vi "AI-Volt.vi"(6 "Slot":T1, 8 "error in":errorcluster, 10 "Mode":string, 11 "CH":string) -> (0 "error out":errorcluster, 3 "data":dbl caption="数据" format="%0.2f")   [LabVIEW 2013]
uses:
  SystemCode/SysControl/Slot.ctl
  <vilib>/DAQmx/read.llb/DAQmx Read (Analog 1D DBL 1Chan NSamp).vi
  SourceCode/GlobalValue.vi
  <vilib>/DAQmx/create/channels.llb/DAQmx Create Channel (AI-Voltage-Basic).vi
  <vilib>/measure/madcrms.llb/Basic Averaged DC-RMS for 1 Chan.vi
  <vilib>/DAQmx/miscellaneous.llb/DAQmx Fill In Error Info.vi
  <vilib>/measure/NI_MAPro.lvlib
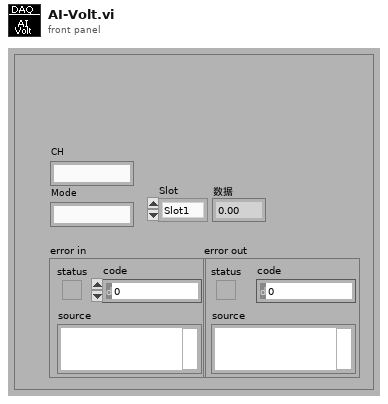
[diagram p1: front panel]
types:
  T1 = typedef "Slot.ctl" = enum16{"Slot1", "Slot2", "Slot3", "Slot4"}
  T2 = typedef "DAQConfig.ctl" = cluster{"DIO":string[][], "AO":string[][], "AI":string[][]}
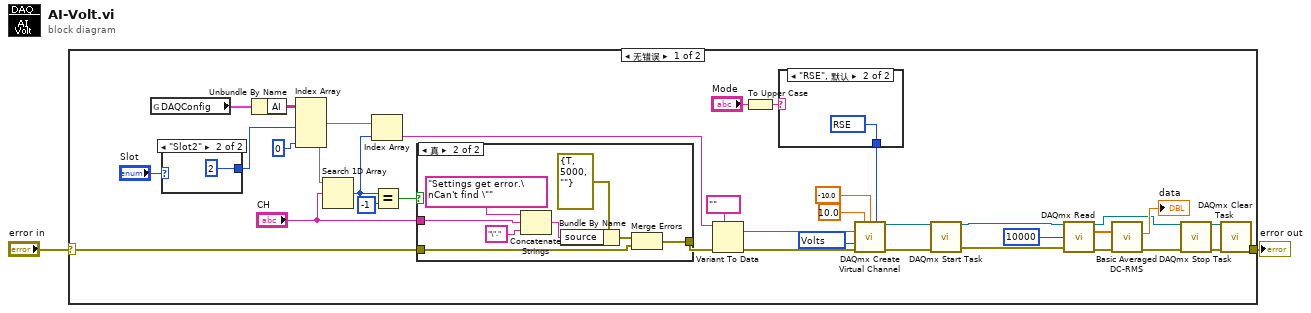
[diagram p0: block diagram]
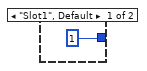
[diagram p2: hidden frame]
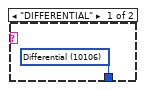
[diagram p3: hidden frame]
diagram:
  n1 = case shown="无错误" "error in" {
    selector: "error in" -> [w22 w52]
    tunnel: [w38 w52] -> w2
    frame No Error {
      w37 = 10348 items=["Volts"=10348, "From Custom Scale"=10065] ("units")
      n2 = global read "GlobalValue.vi" "DAQConfig"() -> (w12:T2)
      n3 = case shown="\"Slot2\"" "Slot" {
        tunnel: [1 ("索引 (行)") 2 ("索引 (行)")] -> w13
        frame "Slot1", Default {
        }
        frame "Slot2" {
        }
      }
      n4 = Unbundle By Name(w12) -> ("AI"=w34:string[][])
      n5 = Index Array(array=w34, index (col) #1=w13, index (col) #2=0 ("索引 (列)")) -> (element #1=w30:string[], element #2=w29:string[])  [unwired: 2 in]
      n6 = Search 1D Array(1D array=w29, element="CH") -> (index of element=w32:i32)  [unwired: 1 in]
      n7 = Index Array(array=w30, index=w32) -> (element=w21:string)
      n8 = Equal?(x=w32, y=-1) -> (x = y?=w28:bool)
      n9 = case shown="真" w28 {
        tunnel: w22 -> [w43 w47]
        tunnel: [w43 w46] -> w23
        tunnel: "CH" -> [_ w45]
        frame False {
        }
        frame True {
          n10 = Concatenate Strings("Settings get error.\nCan't find \"" ("message"), w45, "\"." ("string")) -> (w50:string)
          n11 = Bundle By Name(cluster=errorcluster {"status"=TRUE, "code"=5000, "source"=""} ("error in 1 (no error)"), "source"=w50) -> (w49:errorcluster)
          n12 = Merge Errors(w49, w47) -> (w46:errorcluster)
        }
      }
      n13 = Variant To Data(error in=w23, type=tag "" ("lines"), Variant=w21) -> (data=w25:tag, error out=w24:errorcluster)
      n14 = To Upper Case(1:"Mode") -> (0:w19:string)
      n15 = case shown="\"RSE\", 默认" w19 {
        tunnel: [w41 w42] -> w18
        frame "DIFFERENTIAL" {
          w41 = 10106 items=["default"=-1, "RSE"=10083, "NRSE"=10078, "Differential"=10106, "Pseudodifferential"=12529] ("input terminal configuration")
        }
        frame "RSE", Default {
          w42 = 10083 items=["default"=-1, "RSE"=10083, "NRSE"=10078, "Differential"=10106, "Pseudodifferential"=12529] ("input terminal configuration")
        }
      }
      n16 = call-poly <vilib>:"DAQmx Create Virtual Channel.vi"("maximum value"=10.0, "minimum value"=-10.0, "input terminal configuration"=w18, "physical channels"=w25, "units"=w37, "error in"=w24) -> ("task out"=w10:refnum<k21>, "error out"=w8:errorcluster)  [unwired: 8 in]
      n17 = call <vilib>:"DAQmx Start Task.vi"("task/channels in"=w10, "error in"=w8) -> ("task out"=w9:refnum<k21>, "error out"=w7:errorcluster)  [unwired: 12 in]
      n18 = call-poly <vilib>:"DAQmx Read.vi"("task/channels in"=w9, "number of samples per channel"=10000, "error in"=w7) -> ("task out"=w5:refnum<k21>, "data"=w17:dbl[], "error out"=w16:errorcluster)  [unwired: 10 in]
      n19 = call-poly <vilib>:"Basic Averaged DC-RMS.vi"("error in (no error)"=w16, "signal in"=w17) -> ("error out"=w6:errorcluster, "RMS value"=→"data":dbl)  [unwired: 6 in, 2 out]
      n20 = call <vilib>:"DAQmx Stop Task.vi"("task/channels in"=w5, "error in"=w6) -> ("task out"=w4:refnum<k21>, "error out"=w3:errorcluster)  [unwired: 12 in]
      n21 = call <vilib>:"DAQmx Clear Task.vi"("task in"=w4, "error in"=w3) -> ("error out"=w38:errorcluster)  [unwired: 13 in]
    }
    frame Error {
    }
  }
  "error out" <- w2
